vi "Initialize Mono.vi"(8 "error in (no error)":errorcluster, 11 "IJYCCDReqd In":refnum<k7>) -> (0 "error out":errorcluster, 2 "IJYSystemReqd Out":refnum<k7>, 3 "IJYCCDReqd Out":refnum<k7>)   [LabVIEW 2009]
uses:
  Global/GPIB Numbers.vi
panel:
  # "Broken"
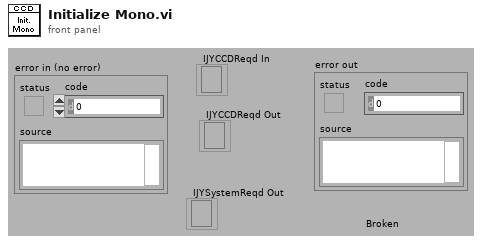
[diagram p1: front panel]
types:
  T1 = typedef "USBCCD Type Def.ctl" = cluster{"Name":string, "Unique ID":string, "Mono Unique ID":string}
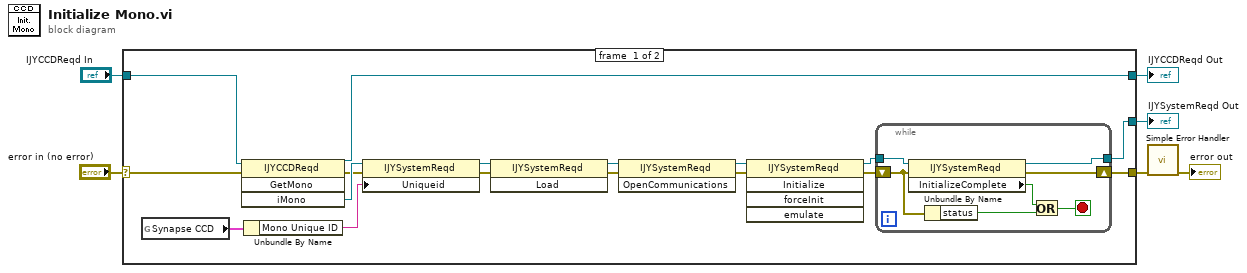
[diagram p0: block diagram]
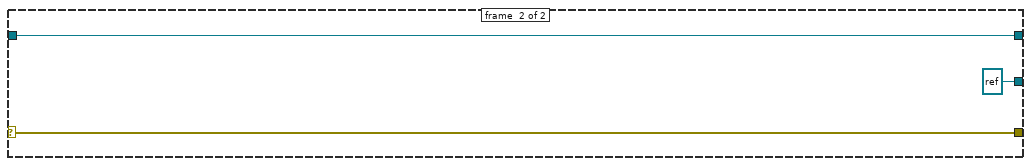
[diagram p2: hidden frame]
diagram:
  n1 = case shown="No Error" "error in (no error)" {
    selector: "error in (no error)" -> [w9 w31]
    tunnel: [w13 w31] -> w4
    tunnel: [w12 refnum<k7> refnum ("IJYSystemReqd")] -> w6
    tunnel: "IJYCCDReqd In" -> [w11 w32]
    tunnel: [w7 w32] -> w1
    frame #0 {
      n2 = global read "GPIB Numbers.vi" "Synapse CCD"() -> (w23:T1)
      n3 = invoke class="IJYCCDReqd" method="GetMono"(reference=w11, error in=w9) -> (reference out=w7:refnum<k7>, error out=w8:errorcluster, "iMono"=w10:refnum<k7>)  [unwired: 2 in, 1 out]
      n4 = Unbundle By Name(w23) -> ("Mono Unique ID"=w22:string)
      n5 = property class="IJYSystemReqd"(reference=w10, error in=w8, "Uniqueid"=w22) -> (reference out=w21:refnum<k7>, error out=w20:errorcluster)
      n6 = invoke class="IJYSystemReqd" method="Load"(reference=w21, error in=w20) -> (reference out=w19:refnum<k7>, error out=w18:errorcluster)  [unwired: 1 in, 1 out]
      n7 = invoke class="IJYSystemReqd" method="OpenCommunications"(reference=w19, error in=w18) -> (reference out=w17:refnum<k7>, error out=w16:errorcluster)  [unwired: 1 in, 1 out]
      n8 = invoke class="IJYSystemReqd" method="Initialize"(reference=w17, error in=w16) -> (reference out=w15:refnum<k7>, error out=w14:errorcluster)  [unwired: 3 in, 3 out]
      n9 = while {
        tunnel: w15 -> [w30]
        tunnel: [w29] -> w12
        shift-right: [w28] -> w13
        shift-left: w14 -> [w27]
        stop <- w24 stop-if-true
        n10 = property class="IJYSystemReqd"(reference=w30, error in=w27) -> (reference out=w29:refnum<k7>, error out=w28:errorcluster, "InitializeComplete"=w25:bool)
        n11 = Unbundle By Name(w27) -> ("status"=w26:bool)
        n12 = Or(x=w25, y=w26) -> (x .or. y?=w24:bool)
      }
    }
    frame #1 {
    }
  }
  "IJYSystemReqd Out" <- w6
  "IJYCCDReqd Out" <- w1
  n13 = call <vilib>:"Simple Error Handler.vi"("error in (no error)"=w4) -> ("error out"=→"error out":errorcluster)  [unwired: 4 in, 4 out]
